vi "PyBoard <-> Spike BLE.vi"() -> ()   [LabVIEW 2019]
uses:
  <userlib>/MicroPython/VIs/uPythonX/uPythonX.xctl
panel:
  in  "uPythonX":T1(xcontrol)
  in  "PyBoard 3":T1(xcontrol)={"Port"="PyBoard - ASRL44::INSTR", "All Code"="# This example demonstrates a simple temperature sensor peripheral.\n#\n# The sensor's local value updates every second, and it will notify\n# any connected central every 10 seconds.\n\nimport bluetooth\nimport random\nimport struct\nimport time\nfrom ble_advertising import advertising_payload\n\nfrom micropython import const\n_IRQ_CENTRAL_CONNECT                 = const(1 << 0)\n_IRQ_CENTRAL_DISCONNECT              = const(1 << 1)\n\n# org.bluetooth.service.environmental_sensing\n_ENV_SENSE_UUID = bluetooth.UUID(0x181A)\n# org.bluetooth.characteristic.temperature\n_TEMP_CHAR = (bluetooth.UUID(0x2A6E), bluetooth.FLAG_READ|bluetooth.FLAG_NOTIFY,)\n_ENV_SENSE_SERVICE = (_ENV_SENSE_UUID, (_TEMP_CHAR,),)\n\n# org.bluetooth.characteristic.gap.appearance.xml\n_ADV_APPEARANCE_GENERIC_THERMOMETER = const(768)\n\nclass BLETemperature:\n    def __init__(self, ble, name='mpy-temp'):\n        self._ble = ble\n        self._ble.active(True)\n        self._ble.irq(handler=self._irq)\n        ((self._handle,),) = self._ble.gatts_register_services((_ENV_SENSE_SERVICE,))\n        self._connections = set()\n        self._payload = advertising_payload(name=name, services=[_ENV_SENSE_UUID], appearance=_ADV_APPEARANCE_GENERIC_THERMOMETER)\n        self._advertise()\n\n    def _irq(self, event, data):\n        # Track connections so we can send notifications.\n        if event == _IRQ_CENTRAL_CONNECT:\n            conn_handle, _, _, = data\n            self._connections.add(conn_handle)\n        elif event == _IRQ_CENTRAL_DISCONNECT:\n            conn_handle, _, _, = data\n            self._connections.remove(conn_handle)\n            # Start advertising again to allow a new connection.\n            self._advertise()\n\n    def set_temperature(self, temp_deg_c, notify=False):\n        # Data is sint16 in degrees Celsius with a resolution of 0.01 degrees Celsius.\n        # Write the local value, ready for a central to read.\n        self._ble.gatts_write(self._handle, struct.pack('<h', int(temp_deg_c * 100)))\n        if notify:\n            for conn_handle in self._connections:\n                # Notify connected centrals to issue a read.\n                self._ble.gatts_notify(conn_handle, self._handle)\n\n    def _advertise(self, interval_us=500000):\n        self._ble.gap_advertise(interval_us, adv_data=self._payload)\n\n\ndef demo():\n    ble = bluetooth.BLE()\n    temp = BLETemperature(ble)\n\n    t = 25\n    i = 0\n\n    while True:\n        # Write every second, notify every 10 seconds.\n        i = (i + 1) % 10\n        temp.set_temperature(t, notify=i == 0)\n        # Random walk the temperature.\n        t += random.uniform(-0.5, 0.5)\n        time.sleep_ms(1000)\n\n\nif __name__ == '__main__':\n    demo()"}
  in  "Spike 2":T1(xcontrol)={"Port"="Spike - ASRL102::INSTR", "All Code"="'''\nhub.ble.mac()  {'mac_addr': '40:BD:32:41:4F:A3'}\npyboard used  mac:    48:4A:30:01:70:42\n'''\n\nimport hub,utime\n\nhub.bluetooth.info()\n\ndef FindIt():\n     hub.ble.scan (5)\n\n     board = -1\n     while board < 0:\n          utime.sleep_ms(100)\n          clients = hub.ble.scan_result()\n#     print(len(clients))\n          i=0\n          for client in clients:\n#               if client['service_id'] ==  '14200126-D700-0032-6670-6C2D64627970':\n               if client['mac_addr'] ==  '48:4A:30:01:98:62':\n                    print(\"found it\")\n                    board = i\n                    break\n               i += 1\n     return board\n\nboard = Findit()\n#print(board)\n\nif (board > 0):\n     p = hub.ble.connect(board)\n     if p:\n          p_info = p.info()\n          print(p_info)\n          p.callback(lambda v: print('got data:', v))\n          p.subscribe()\n\n          p.send('from hub')\n\n          utime.sleep(10)\n          p.unsubscribe()\n          p.disconnect(p_info['index'])\n"}
  in  "PyBoard 2":T1(xcontrol)={"Port"="PyBoard - ASRL44::INSTR", "All Code"="\n'''\nmac address of pybd: b'HJ0\\x01o\\xf2' or 48:4A:01:6F:F2\n     '''\n     '''\nHR_UUID = ubluetooth.UUID(0x180D)\nHR_CHAR = (ubluetooth.UUID(0x2A37), ubluetooth.FLAG_READ | ubluetooth.FLAG_NOTIFY,)\nHR_SERVICE = (HR_UUID, (HR_CHAR,),)\nSERVICES = (HR_SERVICE, )\n(hr,) = bt.gatts_register_services(SERVICES)\n'''\n\nimport bluetooth,utime\n\nble = bluetooth.BLE()\nble.active(True)\n\nLWP_CHAR = (\n    bluetooth.UUID('00001624-1212-EFDE-1623-785FEABCD123'),\n    bluetooth.FLAG_WRITE | bluetooth.FLAG_NOTIFY,\n    # List of descriptors\n    (   \n        # CCCD\n        (bluetooth.UUID(0x2902), bluetooth.FLAG_READ | bluetooth.FLAG_WRITE), \n    )\n)   \nLPF2_SERVICE = (bluetooth.UUID('00001623-1212-EFDE-1623-785FEABCD123'), (LWP_CHAR,))\nALL_SERVICES = (LPF2_SERVICE,)\n\n(lwp_char, lwp_descr), = ble.gatts_register_services(ALL_SERVICES)\n\ndef bt_irq(x, y):\n    print('bt_irq', x, y)\n        \nble.irq(bt_irq)\n\ndef adv_encode_name(name):\n    name = bytes(name, 'ascii')\n    return bytearray((len(name) + 1, 0x09)) + name\n\ndef adv(name):\n    ble.gap_advertise(100_000, adv_data=b'\\x02\\x01\\x06' + adv_encode_name(name))\n\nadv('pybd-lpf2')\n\nutime.sleep(5)   # wait for pyboard to get ready and connect\n\nble.gatts_notify(64, lwp_char, 'from pybd')\n\nble.gatts_read(lwp_char)"}
  in  "PyBoard <> Vernier":T1(xcontrol)={"Port"="PyBoard - ASRL44::INSTR", "All Code"="import ubluetooth, machine, utime,ubinascii\n\ndef ble_cb(event, data):\n     global bt_event,bt_data,devices\n     bt_event = event, data\n     print('ble event:', event, data)\n     \nbt = ubluetooth.BLE()\nbt.active(1)\nbt_event=None\nbt.irq(ble_cb, 0xffff)\n\ndef sync_cmd(f, args, timeout_ms=1000):\n    global bt_event\n    event = []\n    bt_event = None # clear event\n    f(*args) # call function\n    t0 = utime.ticks_ms()\n    while time.ticks_diff(time.ticks_ms(), t0) < timeout_ms:\n        if bt_event is not None:\n             event.append(bt_event)\n             bt_event = None\n        machine.idle() \n    return event\n    #raise OSError('timeout')\n\n# use it like this\nread_result = sync_cmd(bt.gap_scan, (5000), 5000)\nfor i in read_result:\n     print('Addr type: %d mac addr: %s'%(i[1][0],ubinascii.hexlify(i[1][1],':')))\n\nsync_cmd(bt.connect,(1,b'\\x34\\x15\\x13\\x7F\\xD5\\xCC'))\n\nsync_cmd(bt.gap_connect,(1,b'\\xD0\\xCF\\x5E\\x9B\\x46\\x64'))\nb'\\xd0\\xcf^\\x9bFd',\n#bt.connect(2,b'\\x34\\x15\\x13\\x7F\\xD5\\xCC')\n\n#This works for connecting...\nbt.gap_connect(0,b'\\xd0\\xcf^\\x9bFd')\n\nVERNIER_SERVICE = ubluetooth.UUID('19B10000-E8F2-537E-4F6C-D104768A1214')\nVNR_CHAR = (ubluetooth.UUID(0x2A19), ubluetooth.FLAG_NOTIFY|ubluetooth.FLAG_WRITE,)\nbattery_char, = bt.gatts_add_svc(VERNIER_SERVICE, (VNR_CHAR,))\n\n#bt.advertise(100, adv_data=bytearray('\\x02\\x01\\x02\\x0a\\x09pybd-lpf2'))\n\nBATT_UUID = ubluetooth.UUID('19B10000-E8F2-537E-4F6C-D104768A1214')\nBATT_CHAR = (ubluetooth.UUID(0x2A19), ubluetooth.FLAG_WRITE | ubluetooth.FLAG_NOTIFY,)\nBATT_SERVICE = (BATT_UUID, (BATT_CHAR,),)\nTEMP_UUID = ubluetooth.UUID('8e6f0f58-5819-11e6-8b77-86f30ca893d3')\nTEMP_CHAR = (ubluetooth.UUID('8e6f094a-5819-11e6-8b77-86f30ca893d3'), ubluetooth.FLAG_WRITE | ubluetooth.FLAG_NOTIFY,)\nTEMP_SERVICE = (UART_UUID, (TEMP_CHAR,),)\nSERVICES = (BATT_SERVICE, TEMP_SERVICE,)\n( (bat,), (temp,), ) = bt.gatts_register_services(SERVICES)\n\n\nimport bluetooth\nbt = bluetooth.Bluetooth()\nbt.active(True)\n\nVERNIER_SERVICE = bluetooth.UUID('19B10000-E8F2-537E-4F6C-D104768A1214')\nVNR_CHAR = (bluetooth.UUID(0x2A19), bluetooth.FLAG_NOTIFY|bluetooth.FLAG_WRITE,)\nbattery_char, = bt.gatts_add_svc(VERNIER_SERVICE, (VNR_CHAR,))\n\nbt.advertise(100, adv_data=bytearray('\\x02\\x01\\x02\\x0a\\x09pybd-lpf2'))\n\n\n\n#Now to send data from pyboard->hub do:\n\nbt.gatts_notify(lwp_char, 64, 'from pybd')\n\n#Then on pyboard get this data via:\n\nbt.gatts_read(lwp_char)\n\n# You can also register IRQ callbacks on the pyboard for all BLE events, like this:\n\n'''\ndef bt_irq(event, data):\n    print('bt_irq', event, data)\nbt.irq(bt_irq, bluetooth.IRQ_ALL)\n\nhub.ble.rssi(-70)\nhub.ble.scan(1)\nutime.sleep(1)\ndevices = hub.ble.scan_result()\n\n'''\n\nimport time, machine, bluetooth\n\ndef bt_irq(ev, data):\n    global bt_event\n    bt_event = ev, data\nbt = bluetooth.Bluetooth()\nbt.active(1)\nbt.irq(bt_irq, 0xffff)\n\ndef sync_cmd(f, args, timeout_ms=1000):\n    global bt_event\n    bt_event = None # clear event\n    f(*args) # call function\n    t0 = time.ticks_ms()\n    while bt_event is None and time.ticks_diff(time.ticks_ms(), t0) < timeout_ms:\n        if bt_event is not None:\n            return bt_event\n        machine.idle()\n    raise OSError('timeout')\n"}
  in  "Vernier":T1(xcontrol)={"Port"="Spike - ASRL102::INSTR", "All Code"="import hub,utime\n\ndef dump_data(d):\n     print(\"CB 0:\", d)\n\ndef BLEConnect(searchTime):\n     hub.ble.scan(searchTime)\n     starttime = utime.time()\n     p = False \n     reply = False\n\n     while ((utime.time() -starttime) < searchTime):\n          utime.sleep_ms(10)\n          result = hub.ble.scan_result()\n          for client in result:\n#              print(client['mac_addr'])\n#             if client['service_id'] == '19B10000-E8F2-537E-4F6C-D104768A1214':\n               if client['mac_addr'] == 'D0:CF:5E:9B:46:64':\n                    print('found it')\n                    p = hub.ble.connect(loc)\n                    if p:\n                         reply = True\n                         print('connected')\n                         return reply , p\n     return reply , p\n\nhub.bluetooth.info()\nconnected, p = BLEConnect(30)\nif connected:\n     p.callback(dump_data)\n     p.subscribe()\n#     utime.sleep(20)\n#     p.disconnect( p.info()['index']) \n#     print('done')\n\n\nfor line in result:\n     print(line['mac_addr'])\n\n\n-----------------------\nAddress: d0:cf:5e:9b:46:64\nLocal Name: GDX-TMP 0F1054S7\nRSSI: -75\n'''\n{'service_id': '19B10000-E8F2-537E-4F6C-D104768A1214',\n'rssi': -50, 'man_data': b'\\xfd\\x04 \\xff\\xff\\xff', \n'mac_addr': 'C5:F9:CF:6C:87:27', 'man_id': 13320} \n'''\n\n'''     p.send(b'\\x01')\n     utime.sleep(1)\n     p.send(b'\\x00')\n     utime.sleep(1)'''"}
  in  "Arduino":T1(xcontrol)={"Port"="Spike - ASRL102::INSTR", "All Code"="import hub,utime\n\ndef dump_data(d):\n    print(\"CB 0:\", d)\n\ndef BLEConnect(searchTime):\n     hub.ble.scan(searchTime)\n     utime.sleep(searchTime)\n     result = hub.ble.scan_result()\n\n     loc = 0\n     p = False \n     reply = False\n     for client in result:\n#          if client['service_id'] == '19B10000-E8F2-537E-4F6C-D104768A1214':\n          if client['mac_addr'] == 'C5:F9:CF:6C:87:27':\n               print('found it')\n               p = hub.ble.connect(loc)\n               if p:\n                    reply = True\n                    print('connected')\n               break\n          loc += 1\n     return reply, p\n\nhub.bluetooth.info()\nconnected, p = BLEConnect(2)\nif connected:\n     p.callback(dump_data)\n     p.subscribe()\n     utime.sleep(20)\n     p.disconnect( p.info()['index']) \n     print('done')\n\n\n'''\n{'service_id': '19B10000-E8F2-537E-4F6C-D104768A1214',\n  'rssi': -50, 'man_data': b'\\xfd\\x04 \\xff\\xff\\xff', \n  'mac_addr': 'C5:F9:CF:6C:87:27', 'man_id': 13320} \n'''\n\n'''     p.send(b'\\x01')\n     utime.sleep(1)\n     p.send(b'\\x00')\n     utime.sleep(1)'''"}
  in  "PiZero":T1(xcontrol)={"Port"="192.168.1.10", "All Code"="import gatt, threading\n\n# BLE UUID's\nroot_identifier_uuid = '48c5d828-ac2a-442d-97a3-0c9822b04979'\nuart_service_uuid = '6e400001-b5a3-f393-e0a9-e50e24dcca9e'\ntx_characteristic_uuid = '6e400002-b5a3-f393-e0a9-e50e24dcca9e' # Write\nrx_characteristic_uuid = '6e400003-b5a3-f393-e0a9-e50e24dcca9e' # Notify\n\nhub_uuid = '00001623-1212-EFDE-1623-785FEABCD123'\nLWP_CHAR = '00001624-1212-EFDE-1623-785FEABCD123'\n\nclass BluetoothDeviceManager(gatt.DeviceManager):\n     robot = None # root robot device\n\n     def device_discovered(self, device):\n          print(\"[%s] Discovered: %s\" % (device.mac_address, device.alias()))\n          self.stop_discovery() # Stop searching\n          self.robot = RootDevice(mac_address=device.mac_address, manager=self)\n          self.robot.connect()\n\nclass RootDevice(gatt.Device):\n     def connect_succeeded(self):\n          super().connect_succeeded()\n          print(\"[%s] Connected\" % (self.mac_address))\n\n     def connect_failed(self, error):\n          super().connect_failed(error)\n          print(\"[%s] Connection failed: %s\" % (self.mac_address, str(error)))\n\n     def disconnect_succeeded(self):\n          super().disconnect_succeeded()\n          print(\"[%s] Disconnected\" % (self.mac_address))\n\n     def services_resolved(self):\n          super().services_resolved()\n          print(\"[%s] Resolved services\" % (self.mac_address))\n\n          self.uart_service = next(\n          s for s in self.services\n          if s.uuid == uart_service_uuid)\n\n          self.tx_characteristic = next(\n          c for c in self.uart_service.characteristics\n          if c.uuid == tx_characteristic_uuid)\n\n          self.rx_characteristic = next(\n          c for c in self.uart_service.characteristics\n          if c.uuid == rx_characteristic_uuid)\n\n          print(self.tx_characteristic)\n\n          self.rx_characteristic.enable_notifications() # listen to RX messages\n          \n\n     def characteristic_value_updated(self, characteristic, value):\n          message = []\n          type = \"\"\n          for byte in value:\n               message.append(byte)\n#        print (\"Messages from Root:\")\n          if message[0] == 4: type = \"Color Sensor\"\n          if message[0] == 12: type = \"Bumper\"\n          if message[0] == 13: type = \"Light Sensor\"\n          if message[0] == 17: type = \"Touch Sensor\"\n          if message[0] == 20: type = \"Cliff Sensor\"\n\n          print(type, message)\n\n\ndef run():\n     manager = BluetoothDeviceManager(adapter_name = 'hci0')\n     manager.start_discovery(service_uuids=[hub_uuid])\n     thread = threading.Thread(target = manager.run)\n     thread.start()\n     char = \"\"\n     try:\n          while manager.robot is None:\n               pass # wait for a root robot to be discovered\n          print(instructions)\n          while char != \"q\":\n               char = getch() # wait for keyboard input\n               drive_root(char)\n               print(\"Quitting\")\n               manager.stop()\n               manager.robot.disconnect()\n               thread.join()\n     except KeyboardInterrupt:\n          pass\n"}
  in  "Spike":T1(xcontrol)={"Port"="Spike - ASRL102::INSTR", "All Code"="import hub,utime\n\nhub.ble.scan(10)\n\nutime.sleep(10)\nhub.ble.scan_result()\nhub.bluetooth.info()\n\n# wait a few seconds\np = hub.ble.connect(0) # hopefully index 0 is the pyboard, if not you'll have to find the right index via hub.ble.scan_result()\n\n# {'service_id': '232004FD-4200-0032-6670-6C2D64627970', 'rssi': -16, 'man_data': b'\\x00\\x00\\x80\\x98m\\x9a', 'mac_addr': '48:4A:30:01:9A:C2', 'man_id': 227}\n\n# pyboard used  mac:    48:4A:30:01:70:42\np.callback(lambda data:print(data))\np.subscribe()\n\np.send('from hub')\n\np = hub.ble.connect(1)"}
  in  "PyBoard":T1(xcontrol)={"Port"="PyBoard - ASRL44::INSTR", "All Code"="import bluetooth\nbt = bluetooth.Bluetooth()\nbt.active(True)\n\nLPF2_SERVICE = bluetooth.UUID('00001623-1212-EFDE-1623-785FEABCD123')\nLWP_CHAR = (bluetooth.UUID('00001624-1212-EFDE-1623-785FEABCD123'), bluetooth.FLAG_NOTIFY|bluetooth.FLAG_WRITE,)\nlwp_char, = bt.gatts_add_svc(LPF2_SERVICE, (LWP_CHAR,))\n\nbt.advertise(100, adv_data=bytearray('\\x02\\x01\\x02\\x0a\\x09pybd-lpf2'))\n\n\n\n#Now to send data from pyboard->hub do:\n\nbt.gatts_notify(lwp_char, 64, 'from pybd')\n\n#Then on pyboard get this data via:\n\nbt.gatts_read(lwp_char)\n\n# You can also register IRQ callbacks on the pyboard for all BLE events, like this:\n\n'''\ndef bt_irq(event, data):\n    print('bt_irq', event, data)\nbt.irq(bt_irq, bluetooth.IRQ_ALL)\n\n'''"}
  # "Add search - do not do the wait - start the scan, look for the desired mac address or service_id - and then either stop the scan or do not rescan..."
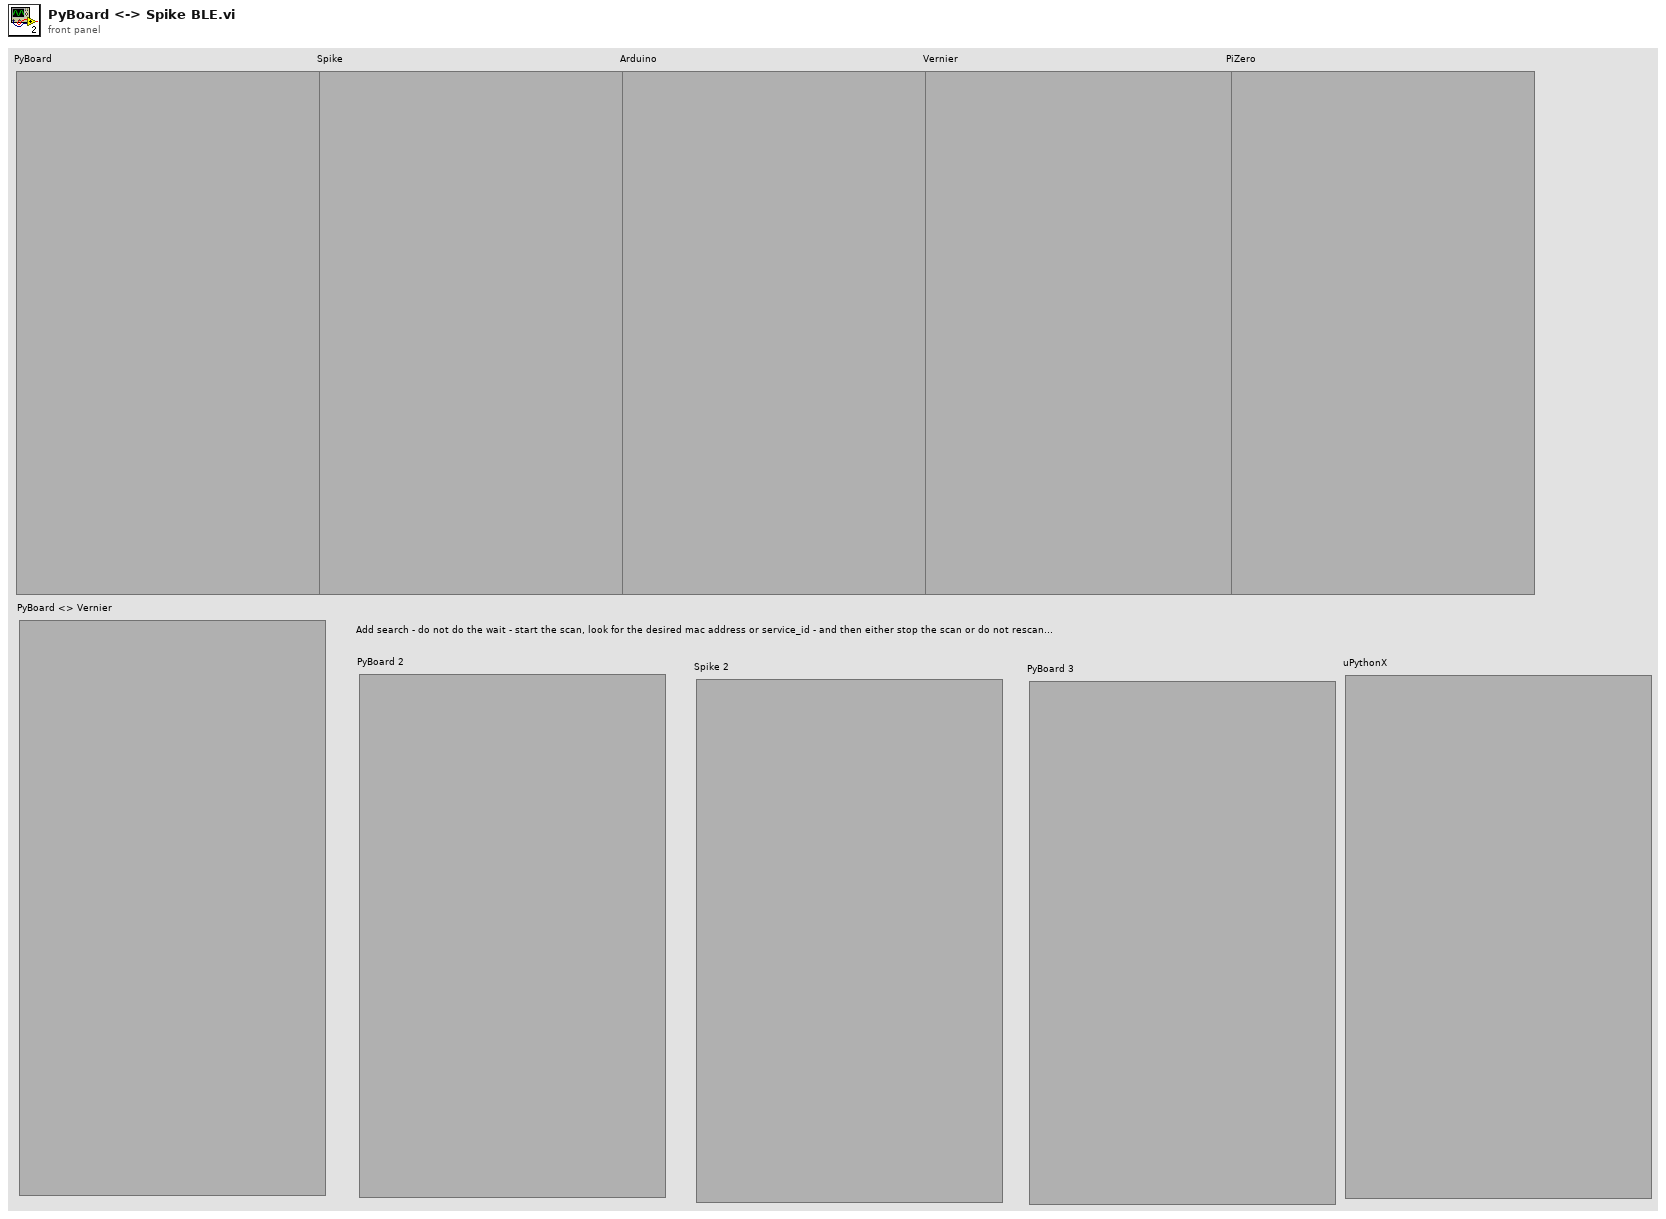
[diagram p1: front panel]
types:
  T1 = cluster{"Port":refnum<visa-resource-name>, "All Code":string}
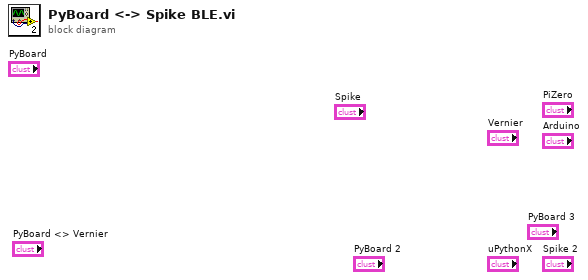
[diagram p0: block diagram]
diagram:
